vi "Read Key.vi"(8 "error in (no error)":errorcluster, 11 "Update Setting in":refnum<class "Update Setting.lvclass">) -> (0 "error out":errorcluster, 2 "Key":string, 3 "Update Setting out":refnum<class "Update Setting.lvclass">)   [LabVIEW 2014, in "Update Setting.lvclass"]
uses:
  Update Setting.lvclass
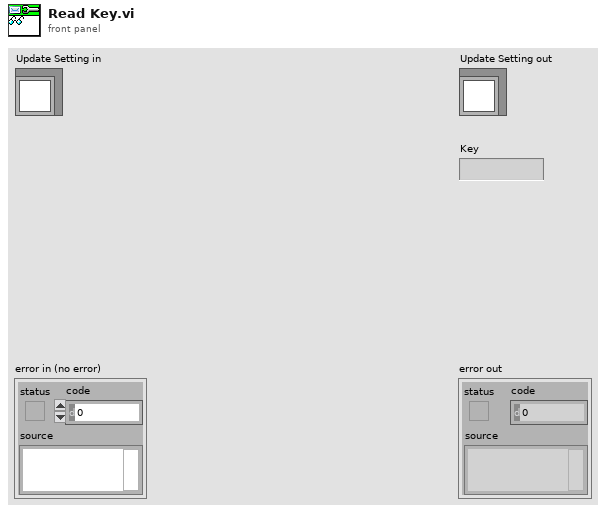
[diagram p1: front panel]
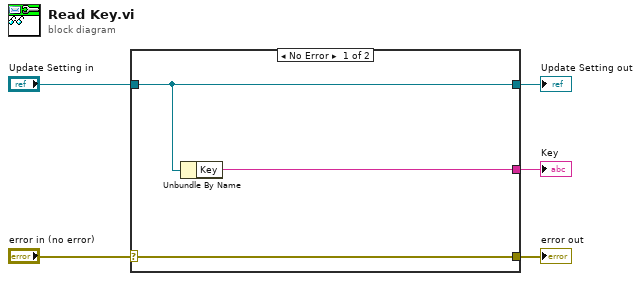
[diagram p0: block diagram]
diagram:
  n1 = case shown="No Error" "error in (no error)" {
    selector: "error in (no error)" -> [w8 w9]
    tunnel: [w8 w9] -> w4
    tunnel: [w7 w10] -> w2
    tunnel: "Update Setting in" -> [w7 w10]
    tunnel: [w6 _] -> w1
    frame No Error {
      n2 = Unbundle By Name(w7) -> ("Key"=w6:string)
    }
    frame Error {
    }
  }
  "error out" <- w4
  "Update Setting out" <- w2
  "Key" <- w1
